vi "SFTP File Type - valid file type - returns file type.vi"(10 "type":T1, 11 "permissions":u32 format="%.0o") -> (0 "error out":errorcluster)   [LabVIEW 2017, in "unit_tests.lvlib"]
uses:
  unit_tests.lvlib
  libssh2/SFTP File Type.ctl
  libssh2/libssh2.lvlib
  <vilib>/PNR/Transparent Assertions/Transparent Assertions/Transparent Assertions.lvlib
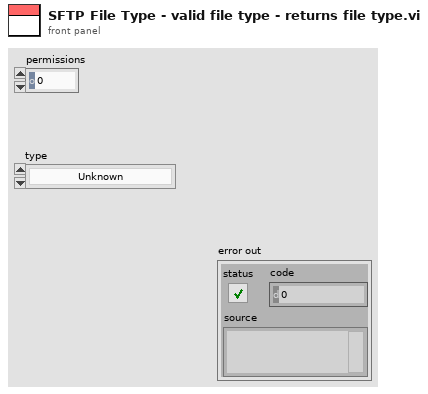
[diagram p1: front panel]
types:
  T1 = typedef "libssh2.lvlib/SFTP File Type.ctl" = enum16{"Unknown", "Named Pipe (FIFO)", "Character Special File", "Directory", "Block Special File", "Regular File", "Symbolic Link", "Socket"}
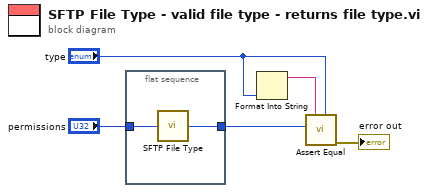
[diagram p0: block diagram]
diagram:
  n1 = flat-sequence {
    tunnel: [w7] -> w4
    tunnel: "permissions" -> [w6]
    frame #0 {
      n2 = call "SFTP File Type.vi"("permissions"=w6) -> ("type"=w7:T1)
    }
  }
  n3 = Format Into String("type") -> (resulting string=w5:string)  [unwired: 3 in, 1 out]
  n4 = call <vilib>:"Assert Equal.vi"("Expected"="type", "Message (\"\")"=w5, "Actual"=w4) -> ("error out"=→"error out":errorcluster)  [unwired: 8 in]
